vi "MC5e Squad_Manager.vi"(7 "Mode":T3=enum."Get Squad", 8 "error in":errorcluster, 9 "Set In":set{T1}(c389), 10 "Squad In (Add/Replace)":T1={"Squad Name"="", "# Soldiers"=1, "Battle Rating"=0, "Flying"=FALSE, "Mounted"=FALSE, "Speed"=3, "Range"=1, "Morale"=0, "Token Image"=variant, "Max Endurance"=10, "Current Endurance"=10, "Size"=enum."Medium", "Space Taken"=1, "Difficult Terrain"=[0, 1, 3, 6, 7], "CR"=1, "Special / Notes"=""} {"CR" items=["1/8", "1/4", "1/2", "1", "2", "3", "4", "5", "6", "7", "8", "9", "10", "11", "12", "13", "14", "15", "16", "17", "18", "19", "20", "21", "22", "23", "24", "25", "26", "27", "28", "29", "30"]}, 11 "index (get/delete)":i32) -> (0 "error out":errorcluster, 1 "set size":i32, 2 "Set":set{T1}(c389), 3 "Squad":T1={"Squad Name"="", "# Soldiers"=1, "Battle Rating"=0, "Flying"=FALSE, "Mounted"=FALSE, "Speed"=3, "Range"=1, "Morale"=0, "Token Image"=variant, "Max Endurance"=10, "Current Endurance"=10, "Size"=enum."Medium", "Space Taken"=1, "Difficult Terrain"=[0, 1, 3, 6, 7], "CR"=1, "Special / Notes"=""} {"CR" items=["1/8", "1/4", "1/2", "1", "2", "3", "4", "5", "6", "7", "8", "9", "10", "11", "12", "13", "14", "15", "16", "17", "18", "19", "20", "21", "22", "23", "24", "25", "26", "27", "28", "29", "30"]})   [LabVIEW 2020]
uses:
  MC5e Squad_Manager_Modes.ctl
  MC5e Squad_Info.ctl
  MC5e Size_Categories.ctl
  MC5e Squad_Set.ctl
panel:
  # "Squads are restricted to one type of soldier (i.e  Archers) and all of the same level.\nIf you want mixed CR or mixed types, use multiple squads."
  # "Squads are restricted to one type of soldier (i.e  Archers) and all of the same level.\nIf you want mixed CR or mixed types, use multiple squads."
  # "Squads are restricted to one type of soldier (i.e  Archers) and all of the same level.\nIf you want mixed CR or mixed types, use multiple squads."
  # "Squads are restricted to one type of soldier (i.e  Archers) and all of the same level.\nIf you want mixed CR or mixed types, use multiple squads."
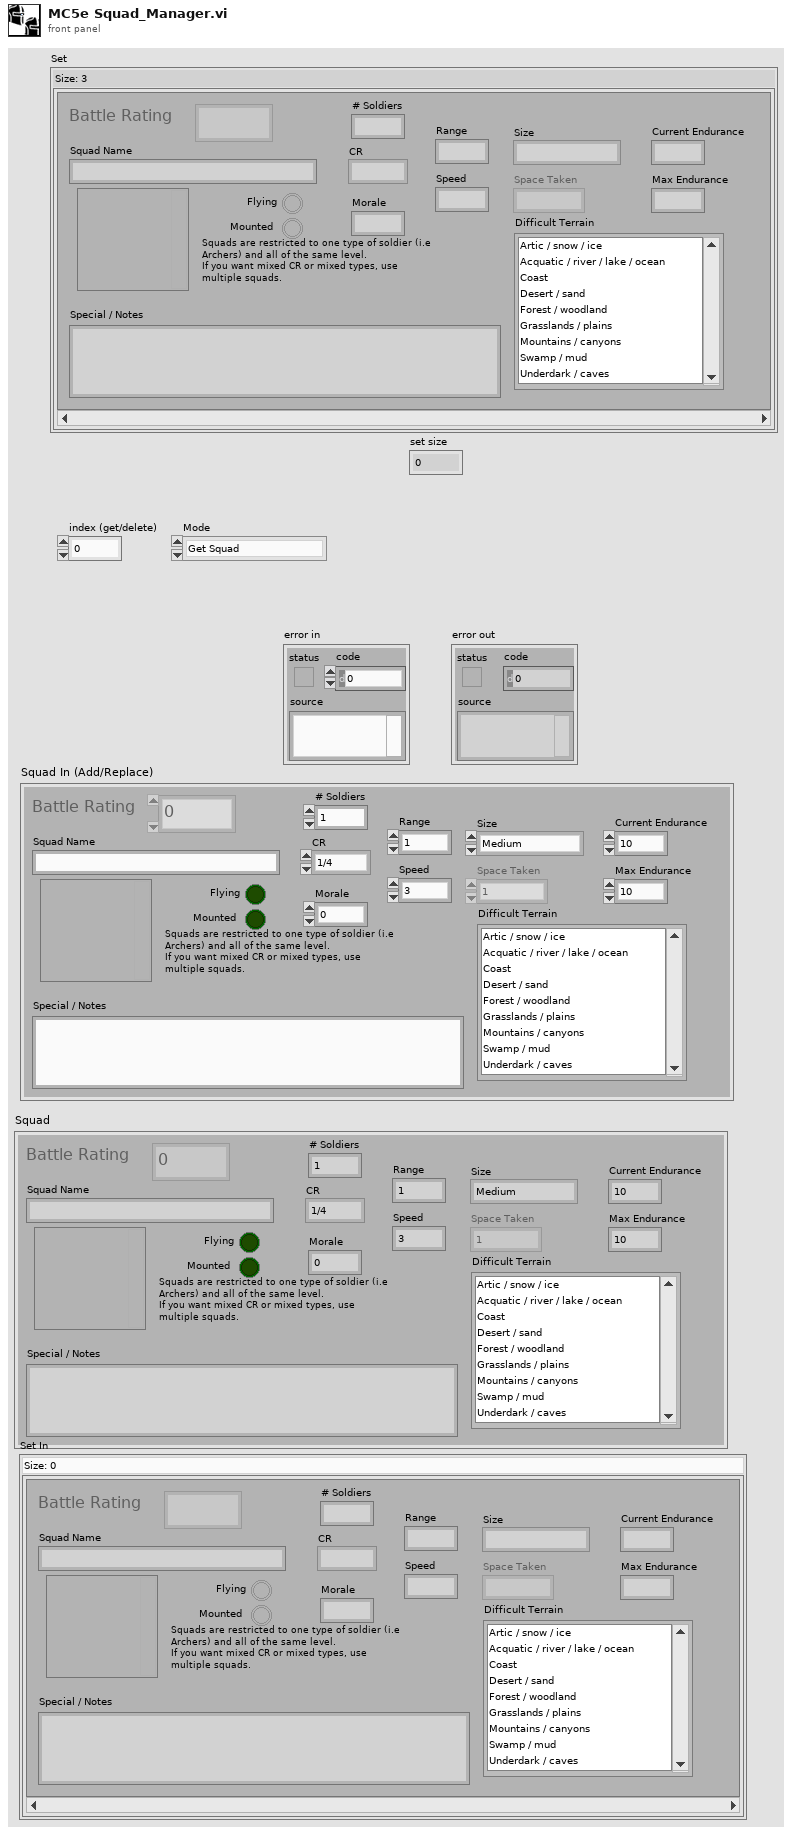
[diagram p1: front panel]
types:
  T1 = typedef "MC5e Squad_Info.ctl" = cluster{"Squad Name":string, "# Soldiers":u16, "Battle Rating":u16, "Flying":bool, "Mounted":bool, "Speed":u16, "Range":u16, "Morale":i32, "Token Image":variant, "Max Endurance":u16, "Current Endurance":i32, "Size":T2, "Space Taken":u16, "Difficult Terrain":i32[], "CR":u16, "Special / Notes":string}
  T2 = typedef "MC5e Size_Categories.ctl" = enum16{"Tiny", "Small", "Medium", "Large", "Huge", "Gargantuan"}
  T3 = typedef "MC5e Squad_Manager_Modes.ctl" = enum16{"Initialize", "Add Squad", "Delete Squad", "Get Squad", "Load Set"}
  T4 = typedef "MC5e Squad_Set.ctl" = set{T1}
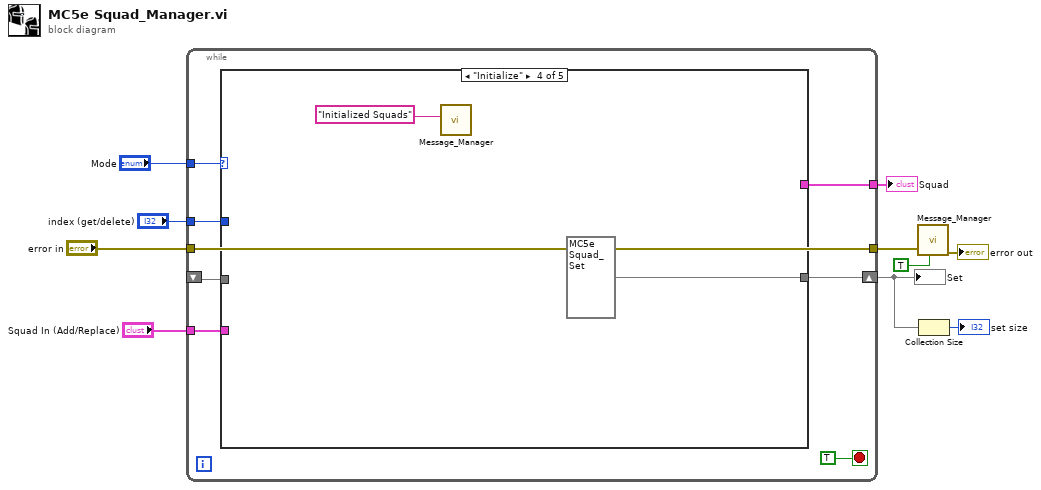
[diagram p0: block diagram]
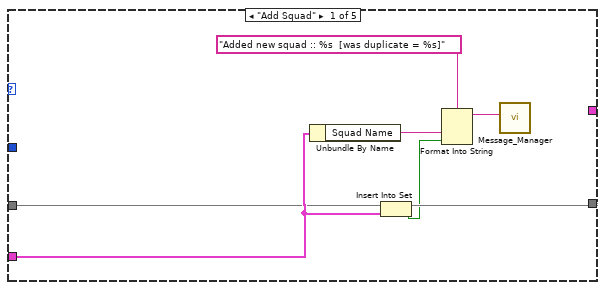
[diagram p2: hidden frame]
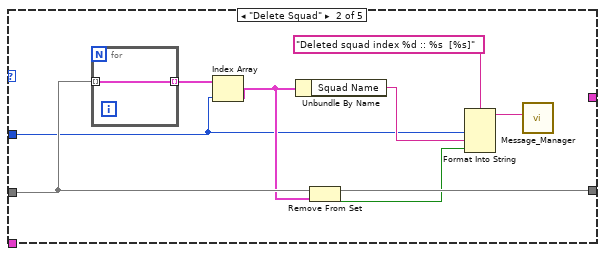
[diagram p3: hidden frame]
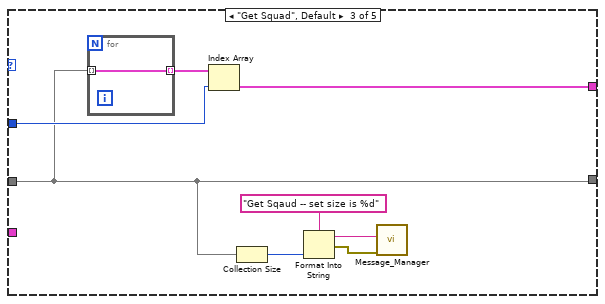
[diagram p4: hidden frame]
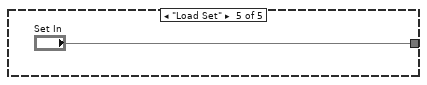
[diagram p5: hidden frame]
diagram:
  n1 = while {
    tunnel: "error in" -> [w12]
    tunnel: "Mode" -> [w17]
    shift-right: [w16] -> w2
    shift-left: _ -> [w15]
    tunnel: "index (get/delete)" -> [w14]
    tunnel: [w13] -> w6
    tunnel: [w12] -> w5
    tunnel: "Squad In (Add/Replace)" -> [w11]
    stop <- TRUE stop-if-true
    n2 = case shown="\"Initialize\"" w17 {
      tunnel: [w25 w32 w39 T4 {} ("Squad List") "Set In"] -> w16
      tunnel: w15 -> [w19 w33 w39 _ _]
      tunnel: w14 -> [_ w27 w41 _ _]
      tunnel: [_ _ w42 _ _] -> w13
      tunnel: w11 -> [w20 _ _ _ _]
      frame "Add Squad" {
        n3 = Unbundle By Name(w20) -> ("Squad Name"=w23:string)
        n4 = Insert Into Set(10:w20, 11:w19) -> (2:w21:bool, 3:w25:set{T1})
        n5 = Format Into String(format string="Added new squad :: %s  [was duplicate = %s]", w23, w21) -> (resulting string=w22:string)  [unwired: 2 in, 1 out]
        n6 = call "Message_Manager.vi"("New Entry"=w22) -> ()  [unwired: 6 in, 5 out]
      }
      frame "Delete Squad" {
        n7 = for {
          tunnel: [w35] -> w34 mode=indexing
          tunnel: w33 -> [w35] mode=indexing
        }
        n8 = Index Array(array=w34, index=w27) -> (element=w28:T1)
        n9 = Unbundle By Name(w28) -> ("Squad Name"=w30:string)
        n10 = Remove From Set(10:w28, 11:w33) -> (2:w26:bool, 3:w32:set{T1})
        n11 = Format Into String(format string="Deleted squad index %d :: %s  [%s]", w27, w30, w26) -> (resulting string=w29:string)  [unwired: 2 in, 1 out]
        n12 = call "Message_Manager.vi"("New Entry"=w29) -> ()  [unwired: 6 in, 5 out]
      }
      frame "Get Squad", Default {
        n13 = for {
          tunnel: [w44] -> w43 mode=indexing
          tunnel: w39 -> [w44] mode=indexing
        }
        n14 = Index Array(array=w43, index=w41) -> (element=w42:T1)
        n15 = Collection Size(1:w39) -> (0:w38:i32)
        n16 = Format Into String(format string="Get Sqaud -- set size is %d", w38) -> (resulting string=w37:string, error out=w36:errorcluster)  [unwired: 2 in]
        n17 = call "Message_Manager.vi"("error in"=w36, "New Entry"=w37) -> ()  [unwired: 5 in, 5 out]
      }
      frame "Initialize" {
        n18 = call "Message_Manager.vi"("New Entry"="Initialized Squads" ("format string")) -> ()  [unwired: 6 in, 5 out]
      }
      frame "Load Set" {
      }
    }
  }
  "Squad" <- w6
  "Set" <- w2
  n19 = call "Message_Manager.vi"("Log only on Err"=TRUE, "error in"=w5) -> ("error out"=→"error out":errorcluster)  [unwired: 5 in, 4 out]
  n20 = Collection Size(1:w2) -> (0:→"set size":i32)
